vi "flipHolo.vi"(8 "error in (no error)":errorcluster, 10 "flip_option":string, 11 "Image in":T1) -> (0 "error out":errorcluster, 3 "Image out":T1)   [LabVIEW 2023]
uses:
  <vilib>/vision/Image Controls.llb/IMAQ Image.ctl
  <vilib>/vision/NI_Vision_Development_Module.lvlib
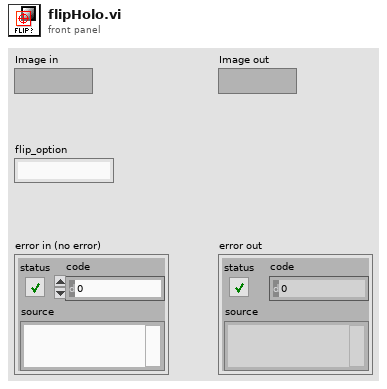
[diagram p1: front panel]
types:
  T1 = typedef "IMAQ Image.ctl" = refnum<image>
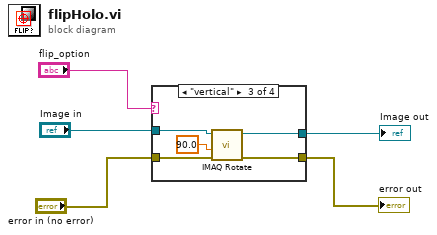
[diagram p0: block diagram]
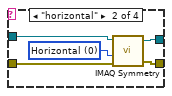
[diagram p3: hidden frame]
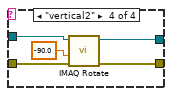
[diagram p4: hidden frame]
diagram:
  n1 = case shown="\"vertical\"" "flip_option" {
    tunnel: "error in (no error)" -> [w6 w12 w16 w20]
    tunnel: [w6 w11 w17 w19] -> w2
    tunnel: "Image in" -> [w7 w10 w15 w21]
    tunnel: [w7 w9 w13 w18] -> w5
    frame "no flip", Default {
    }
    frame "horizontal" {
      w8 = u32 0 items=["Horizontal", "Vertical", "Central", "1st Diagonal", "2nd Diagonal"] ("Type of Symmetry")
      n2 = call "IMAQ Symmetry"("error in (no error)"=w12, "Type of Symmetry"=w8, "Image Src"=w10) -> ("error out"=w11:errorcluster, "Image Dst Out"=w9:T1)  [unwired: 2 in]
    }
    frame "vertical" {
      n3 = call "IMAQ Rotate"("error in (no error)"=w16, "Angle (degrees)"=sgl 90.0, "Image Src"=w15) -> ("error out"=w17:errorcluster, "Image Dst Out"=w13:T1)  [unwired: 7 in]
    }
    frame "vertical2" {
      n4 = call "IMAQ Rotate"("error in (no error)"=w20, "Angle (degrees)"=sgl -90.0, "Image Src"=w21) -> ("error out"=w19:errorcluster, "Image Dst Out"=w18:T1)  [unwired: 7 in]
    }
  }
  "Image out" <- w5
  "error out" <- w2
